vi "tm481_wview.vi"() -> ()   [LabVIEW 2011]
panel:
  out "Current Timestamp":dbl
  out "Image B":u16[][](graph) caption="Image"
  out "Image A":u16[][](graph) caption="Image"
  in  "Vertical Width":i32=512
  in  "Horizontal Width":i32=512
  in  "Vertical Offset B":i32=64
  in  "Horizontal Offset B":i32=256
  in  "Vertical Offset A":i32=128
  in  "Horizontal Offset A":i32=512
  out "Frames Per Second":dbl
  in  "Quit":bool
  out "Error Out":errorcluster {"code" format="%.0x"}
  # "This is just a simple example\nof how to setup a camera for\na W-View application with\na Flash4.0 LT"
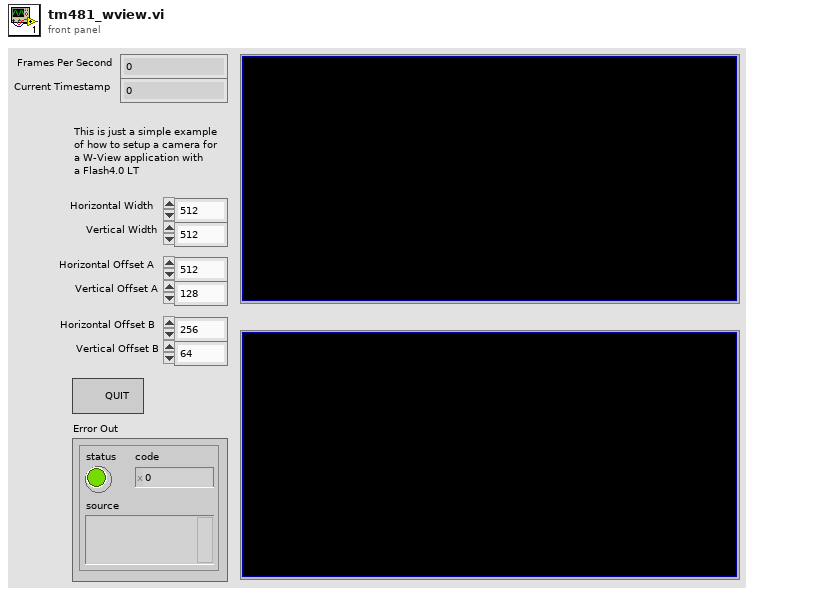
[diagram p1: front panel]
types:
  T1 = cluster{"Horizontal Offset A":i32, "Vertical Offset A":i32, "Horizontal Offset B":i32, "Vertical Offset B":i32, "Horizontal Width":i32, "Vertical Width":i32}
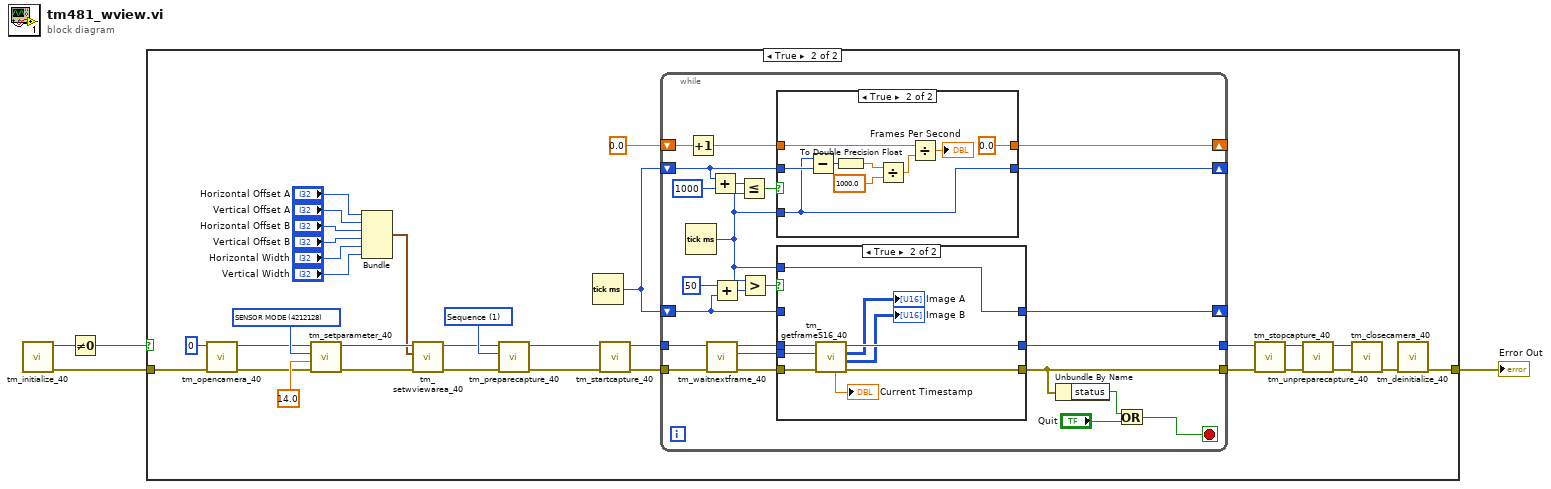
[diagram p0: block diagram]
diagram:
  n1 = call <userlib>:"tm_initialize_40.vi"() -> ("error out"=w1:errorcluster, "Number Of Cameras"=w2:u32)  [unwired: 8 in, 2 out]
  n2 = Not Equal To 0?(x=w2) -> (x != 0?=w4:bool)
  n3 = case shown="True" w4 {
    tunnel: w1 -> [w5 w37]
    tunnel: [w5 w34] -> w3
    frame False {
    }
    frame True {
      w19 = u32 4212128 items=["SENSOR MODE"=4212128, "CCD MODE"=4212384, "READOUT MODE"=4211872, "ACTIVE VIEW INDEX"=4343136, "BITS PER CHANNEL"=4342976, "IMAGE PIXEL TYPE"=4343296, "BINNING"=4215968, "EXPOSURE TIME"=2049184, "CONTRAST GAIN"=3163312, "CONTRAST OFFSET"=3163328, "LIGHT MODE"=2114720, "SENSITIVITY"=2114992, "PHOTON IMAGING MODE"=2115200, "HIGH DYNAMIC RANGE MODE"=3163360, "WHITE BALANCE"=3163568, "TEMPERATURE"=2115232, "TEMPERATURE TARGET"=2115264, "SENSOR COOLER FAN"=2115296, "LINEBUNDLE HEIGHT"=4212192, "MECHANICAL SHUTTER"=2115488, "BACK FOCUS POSITION"=8422304, "TRIGGER CONNECTOR"=1066432, "TRIGGER SOURCE"=1066144, "OUTPUT TRIGGER SOURCE"=1852576, "TRIGGER GLOBAL EXPOSURE"=2049680, "FIRST TRIGGER BEHAVIOR"=2049696, "CHANNEL SYNC"=1852352, "READOUT DIRECTION"=4211904, "PRE HSYNC COUNT"=1852704, "INTERNAL LINE SPEED"=4191408, "INTERNAL LINE INTERVAL"=4191424] ("Parameter")
      w25 = 1 items=["Snap", "Sequence"] ("Capture mode")
      n4 = call <userlib>:"tm_opencamera_40.vi"("error in (no error)"=w37, "Camera Index"=u32 0) -> ("error out"=w17:errorcluster, "Handle out"=w18:u32)  [unwired: 7 in, 1 out]
      n5 = call <userlib>:"tm_setparameter_40.vi"("error in (no error)"=w17, "Value in"=14.0, "Parameter"=w19, "Handle in"=w18) -> ("error out"=w15:errorcluster, "Handle out"=w16:u32)  [unwired: 6 in]
      n6 = Bundle("Horizontal Offset A"="Horizontal Offset A", "Vertical Offset A"="Vertical Offset A", "Horizontal Offset B"="Horizontal Offset B", "Vertical Offset B"="Vertical Offset B", "Horizontal Width"="Horizontal Width", "Vertical Width"="Vertical Width") -> (w12:T1)  [unwired: 1 in]
      n7 = call <userlib>:"tm_setwviewarea_40.vi"("error in (no error)"=w15, "Sub Region"=w12, "Handle in"=w16) -> ("error out"=w14:errorcluster, "Handle out"=w13:u32)  [unwired: 7 in]
      n8 = call <userlib>:"tm_preparecapture_40.vi"("error in (no error)"=w14, "Capture mode"=w25, "Handle in"=w13) -> ("error out"=w23:errorcluster, "Handle out"=w24:u32)  [unwired: 5 in, 2 out]
      n9 = Tick Count (ms)() -> (millisecond timer value=w21:u32)
      n10 = call <userlib>:"tm_startcapture_40.vi"("error in (no error)"=w23, "Handle in"=w24) -> ("error out"=w26:errorcluster, "Handle out"=w27:u32)  [unwired: 8 in]
      n11 = while {
        tunnel: [w40] -> w30
        tunnel: [w41] -> w31
        tunnel: w27 -> [w58]
        tunnel: w26 -> [w59]
        shift-right: [w56] -> _
        shift-left: w21 -> [w53]
        shift-right: [w57] -> _
        shift-left: 0.0 -> [w50]
        shift-right: [w39] -> _
        shift-left: w21 -> [w42]
        stop <- w38 stop-if-true
        n12 = Tick Count (ms)() -> (millisecond timer value=w43:u32)
        n13 = Increment(x=w50) -> (x+1=w51:dbl)
        n14 = call <userlib>:"tm_waitnextframe_40.vi"("error in (no error)"=w59, "Handle in"=w58) -> ("error out"=w48:errorcluster, "Frame Index"=w47:i32, "Handle out"=w49:u32)  [unwired: 6 in, 1 out]
        n15 = Add(x=w53, y=u32 1000) -> (x+y=w55:u32)
        n16 = Add(x=u32 50, y=w42) -> (x+y=w45:u32)
        n17 = Less Or Equal?(x=w55, y=w43) -> (x <= y?=w52:bool)
        n18 = Greater?(x=w43, y=w45) -> (0:w44:bool)
        n19 = case shown="True" w52 {
          tunnel: w53 -> [w75 w78]
          tunnel: [w75 w76] -> w56
          tunnel: w51 -> [w74 w82]
          tunnel: w43 -> [_ w76]
          tunnel: [w74 0.0] -> w57
          frame False {
          }
          frame True {
            n20 = Subtract(x=w76, y=w78) -> (x-y=w77:u32)
            n21 = To Double Precision Float(number=w77) -> (double precision float=w84:dbl)
            n22 = Divide(x=w84, y=1000.0) -> (x/y=w81:dbl)
            n23 = Divide(x=w82, y=w81) -> (x/y=→"Frames Per Second":dbl)
          }
        }
        n24 = case shown="True" w44 {
          tunnel: w49 -> [w64 w70]
          tunnel: w48 -> [w63 w72]
          tunnel: w47 -> [_ w71]
          tunnel: w42 -> [w62 _]
          tunnel: w43 -> [_ w73]
          tunnel: [w64 w69] -> w40
          tunnel: [w63 w66] -> w41
          tunnel: [w62 w73] -> w39
          frame False {
          }
          frame True {
            n25 = call <userlib>:"tm_getframeS16_40.vi"("error in (no error)"=w72, "Frame Index"=w71, "Handle in"=w70) -> ("error out"=w66:errorcluster, "Data B"=→"Image B":u16[][], "Data A"=→"Image A":u16[][], "Handle out"=w69:u32, "Timestamp"=→"Current Timestamp":dbl)  [unwired: 4 in]
          }
        }
        n26 = Unbundle By Name(w41) -> ("status"=w61:bool)
        n27 = Or(x=w61, y="Quit") -> (x .or. y?=w38:bool)
      }
      n28 = call <userlib>:"tm_stopcapture_40.vi"("error in (no error)"=w31, "Handle in"=w30) -> ("error out"=w28:errorcluster, "Handle out"=w29:u32)  [unwired: 8 in]
      n29 = call <userlib>:"tm_unpreparecapture_40.vi"("error in (no error)"=w28, "Handle in"=w29) -> ("error out"=w33:errorcluster, "Handle out"=w32:u32)  [unwired: 8 in]
      n30 = call <userlib>:"tm_closecamera_40.vi"("error in (no error)"=w33, "Handle in"=w32) -> ("error out"=w35:errorcluster)  [unwired: 9 in]
      n31 = call <userlib>:"tm_deinitialize_40.vi"("error in (no error)"=w35) -> ("error out"=w34:errorcluster)  [unwired: 10 in]
    }
  }
  "Error Out" <- w3
